vi "Read Image (iSUB) (SubVI).vi"(0 "FPGA REF (iSUB)":T2, 2 "Send":bool=TRUE, 3 "Image Size":T3 {"Width" step=8; "Height" step=8}) -> (4 "N Compressed Bits":u32, 6 "Frame #":u32, 10 "Disk Data":T1, 14 "Display?":bool, 15 "Display Image":u64[](array[numeric]))   [LabVIEW 2015]
uses:
  <vilib>/rvi/interface/nirviMethod/nirviMethod.xnode
  <vilib>/FPGAPlugInAG/Dynamic/niLvFpga_ReadFifo_Dynamic.vi
  <vilib>/rvi/errors/niLvFpgaMergeErrorWithErrorCode.vi
  Controls (HOST)/Data to Disk Bundle.ctl
  Controls (HOST)/FPGA REF (iSUB).ctl
  Controls (HOST)/Image Size.ctl
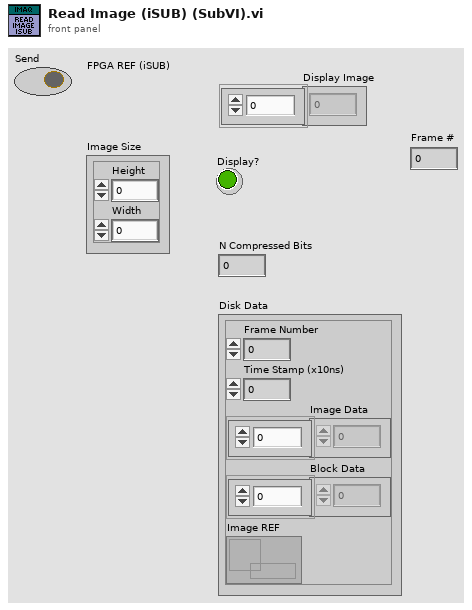
[diagram p1: front panel]
types:
  T1 = typedef "Data to Disk Bundle.ctl" = cluster{"Frame Number":u64, "Time Stamp (x10ns)":u64, "Image Data":u64[], "Block Data":u64[], "Image REF":refnum<data-value>}
  T2 = typedef "FPGA REF (iSUB).ctl" = refnum<k20>
  T3 = typedef "Image Size.ctl" = cluster{"Height":u16, "Width":u16}
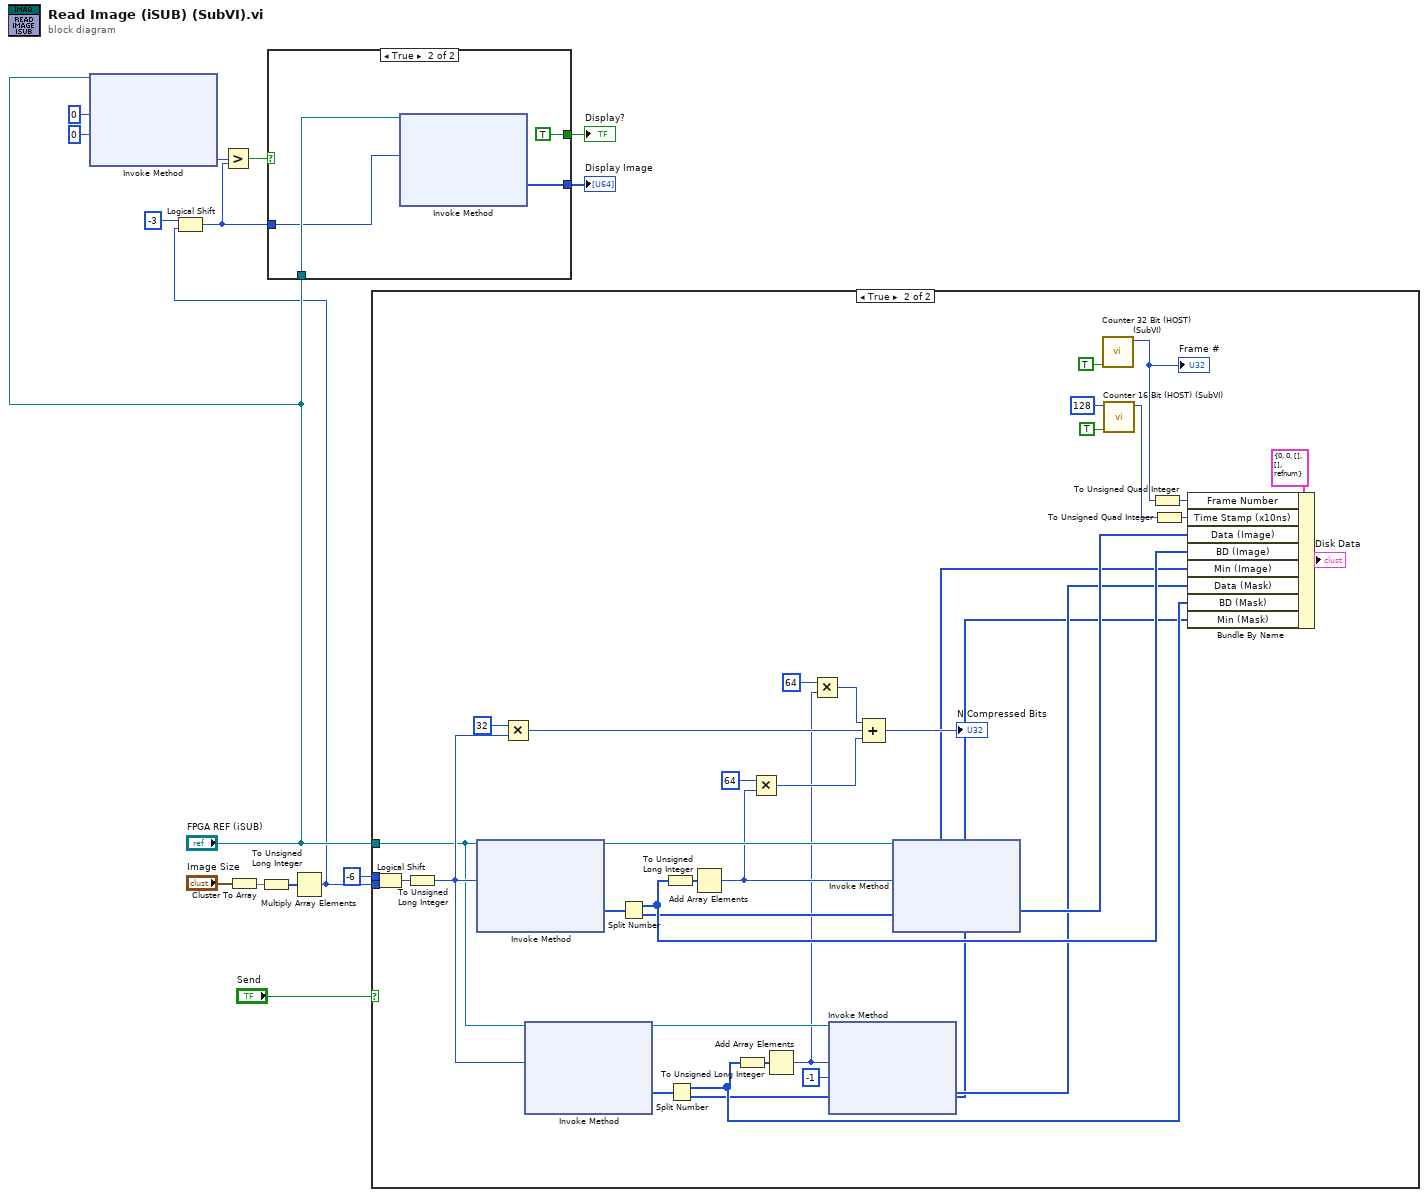
[diagram p0: block diagram]
diagram:
  n1 = xnode "Invoke Method"("FPGA VI Reference In"="FPGA REF (iSUB)", "Number of Elements"=u32 0, "Timeout (ms)"=0) -> ("Elements Remaining"=w7:u32)  [unwired: 1 in, 3 out]
  n2 = Cluster To Array(cluster="Image Size") -> (array=w15:u16[])
  n3 = To Unsigned Long Integer(number=w15) -> (unsigned 32bit integer=w12:u32[])
  n4 = Multiply Array Elements(1:w12) -> (0:w2:u32)
  n5 = Logical Shift(y=i16 -3, x=w2) -> (x << y=w1:u32)
  n6 = Greater?(x=w7, y=w1) -> (0:w8:bool)
  n7 = case shown="True" w8 {
    tunnel: "FPGA REF (iSUB)" -> [_ w19]
    tunnel: [_ w18] -> w11
    tunnel: [_ TRUE] -> w10
    tunnel: w1 -> [_ w16]
    frame False {
    }
    frame True {
      n8 = xnode "Invoke Method"("FPGA VI Reference In"=w19, "Number of Elements"=w16) -> ("Data"=w18:u64[])  [unwired: 2 in, 3 out]
    }
  }
  "Display Image" <- w11
  "Display?" <- w10
  n9 = case shown="True" "Send" {
    tunnel: i16 -6 ("y") -> [_ w55]
    tunnel: w2 -> [_ w50]
    tunnel: "FPGA REF (iSUB)" -> [_ w20]
    frame False {
    }
    frame True {
      n10 = Logical Shift(y=w55, x=w50) -> (x << y=w54:u32)
      n11 = To Unsigned Long Integer(number=w54) -> (unsigned 32bit integer=w28:u32)
      n12 = xnode "Invoke Method"("FPGA VI Reference In"=w20, "Number of Elements"=w28) -> ("FPGA VI Reference Out"=w53:T2, "Data"=w52:u16[])  [unwired: 2 in, 2 out]
      n13 = Multiply(x=u32 32, y=w28) -> (x*y=w46:u32)
      n14 = xnode "Invoke Method"("FPGA VI Reference In"=w20, "Number of Elements"=w28) -> ("FPGA VI Reference Out"=w29:T2, "Data"=w30:u16[])  [unwired: 2 in, 2 out]
      n15 = Split Number(x=w52) -> (hi(x)=w34:u8[], lo(x)=w33:u8[])
      n16 = To Unsigned Long Integer(number=w34) -> (unsigned 32bit integer=w51:u32[])
      n17 = Split Number(x=w30) -> (hi(x)=w26:u8[], lo(x)=w25:u8[])
      n18 = Add Array Elements(numeric array=w51) -> (sum=w47:u32)
      n19 = To Unsigned Long Integer(number=w26) -> (unsigned 32bit integer=w31:u32[])
      n20 = Multiply(x=u32 64, y=w47) -> (x*y=w45:u32)
      n21 = Add Array Elements(numeric array=w31) -> (sum=w22:u32)
      n22 = Multiply(x=u32 64, y=w22) -> (x*y=w21:u32)
      n23 = xnode "Invoke Method"("FPGA VI Reference In"=w29, "Number of Elements"=w22, "Timeout (ms)"=-1) -> ("Data"=w27:u64[])  [unwired: 1 in, 3 out]
      n24 = Compound Arithmetic op=ADD(w21, w46, w45) -> (→"N Compressed Bits":u32)
      n25 = xnode "Invoke Method"("FPGA VI Reference In"=w53, "Number of Elements"=w47) -> ("Data"=w35:u64[])  [unwired: 2 in, 3 out]
      n26 = call "Counter 32 Bit (HOST) (SubVI).vi"("Enable"=TRUE) -> ("Count"=w37:u32)  [unwired: 8 in, 2 out]
      "Frame #" <- w37
      n27 = call "Counter 16 Bit (HOST) (SubVI).vi"("Enable"=TRUE, "Max. Count"=u16 128) -> ("Count"=w40:u16)  [unwired: 7 in, 2 out]
      n28 = To Unsigned Quad Integer(1:w37) -> (0:w36:u64)
      n29 = To Unsigned Quad Integer(1:w40) -> (0:w39:u64)
      n30 = Bundle By Name(cluster=T1 {"Frame Number"=0, "Time Stamp (x10ns)"=0, "Image Data"=[], "Block Data"=[], "Image REF"=refnum}, "Frame Number"=w36, "Time Stamp (x10ns)"=w39, "Data (Image)"=w35, "BD (Image)"=w34, "Min (Image)"=w33, "Data (Mask)"=w27, "BD (Mask)"=w26, "Min (Mask)"=w25) -> (→"Disk Data":T1)
    }
  }
